vi "Run All Tests.vi"() -> ()   [LabVIEW 2013]
panel:
  out "error out":errorcluster
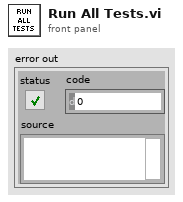
[diagram p1: front panel]
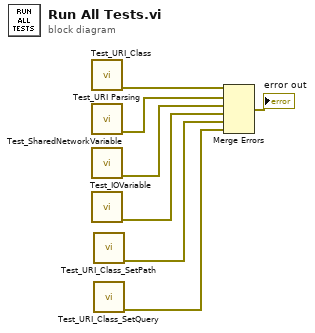
[diagram p0: block diagram]
diagram:
  n1 = call "Test_URI_Class.vi"() -> ("error out"=w7:errorcluster)  [unwired: 11 in]
  n2 = call "Test_URI Parsing.vi"() -> ("error out"=w6:errorcluster)  [unwired: 11 in]
  n3 = call "Test_SharedNetworkVariable.vi"() -> ("error out"=w5:errorcluster)  [unwired: 11 in]
  n4 = call "Test_IOVariable.vi"() -> ("error out"=w4:errorcluster)  [unwired: 11 in]
  n5 = call "Test_URI_Class_SetPath.vi"() -> ("error out"=w2:errorcluster)  [unwired: 11 in]
  n6 = call "Test_URI_Class_SetQuery.vi"() -> ("error out"=w1:errorcluster)  [unwired: 11 in]
  n7 = Merge Errors(w7, w6, w5, w4, w2, w1) -> (→"error out":errorcluster)
